vi "addDevices.vi"(0 "IDevice in":refnum<class "IDevice.lvclass">, 2 "Connection Arguments in":T1(c390), 3 "Error Codes in":map{string, refnum<class "IInteger.lvclass">}(c390), 4 "Error Infos in":map{string, refnum<class "IErrorInfo.lvclass">}(c390), 5 "error in (no error)":errorcluster) -> (14 "IDevice out":refnum<class "IDevice.lvclass">, 15 "Devices out":map{string, refnum<class "IDevice.lvclass">}(c390), 16 "Connection Arguments out":T1(c390), 17 "Error Codes out":map{string, refnum<class "IInteger.lvclass">}(c390), 18 "Error Infos out":map{string, refnum<class "IErrorInfo.lvclass">}(c390), 19 "error out":errorcluster)   [LabVIEW 2022 SP3, in "openDAQ.lvlib" / "IBaseObject.lvlib" / "IPropertyObject.lvlib" / "IComponent.lvlib" / "IFolder.lvlib" / "IDevice.lvlib" / "IDevice.lvclass"]
uses:
  <instrlib>/openDAQ/Public/Classes/IDevice/IDevice.lvclass
  <instrlib>/openDAQ/Public/Classes/IDevice/IDevice.lvclass/IDevice.ctl
  <instrlib>/openDAQ/Public/Classes/daqCoreTypes/IDict/IDict.lvclass
  <instrlib>/openDAQ/Binaries/Windows/x86/copendaq32.dll
  <instrlib>/openDAQ/Public/Classes/daqUtils/daqUtils.lvlib
  <instrlib>/openDAQ/Public/Classes/daqCoreTypes/IDict/Polymorphic/getValueList/getDeviceValueList.vi
  <instrlib>/openDAQ/Public/Classes/daqCoreTypes/IDict/Polymorphic/getKeyList/getStringKeyList.vi
  <instrlib>/openDAQ/Public/Classes/daqCoreTypes/IInteger/IInteger.lvclass
  <instrlib>/openDAQ/Public/Classes/IPropertyObject/IPropertyObject.lvclass
  <instrlib>/openDAQ/Public/Classes/IErrorInfo/IErrorInfo.lvclass
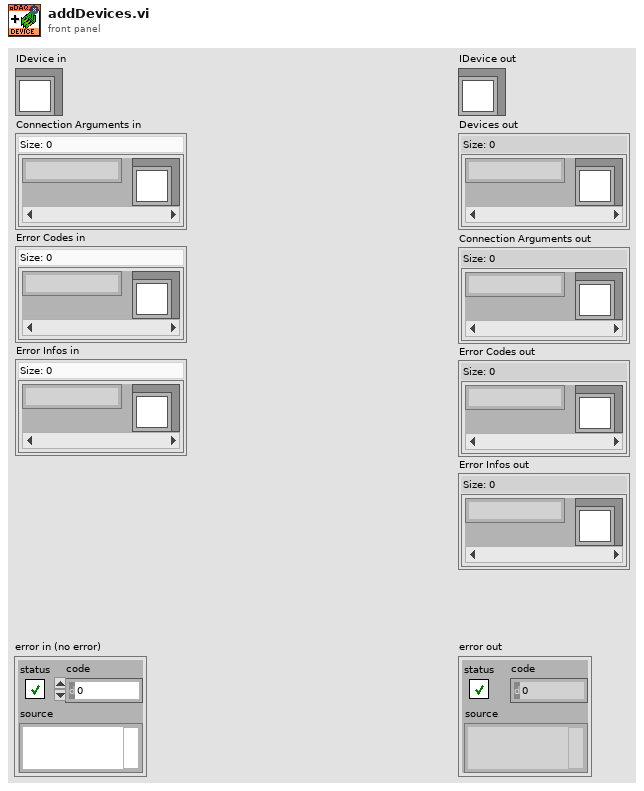
[diagram p1: front panel]
types:
  T1 = map{string, refnum<class "IPropertyObject.lvclass">}
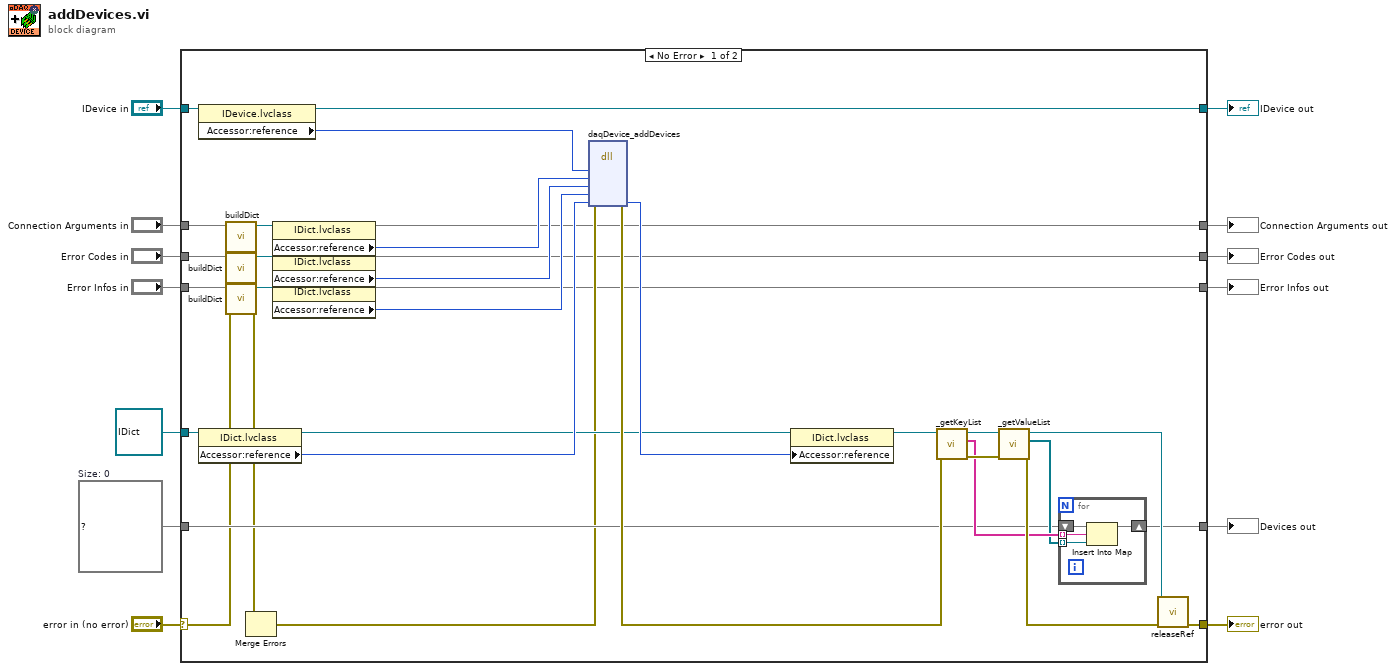
[diagram p0: block diagram]
diagram:
  w8 = map{string, refnum<class "IDevice.lvclass">} {}  # Size: 0
  n1 = case shown="No Error" "error in (no error)" {
    selector: "error in (no error)" -> [w27 w55]
    tunnel: [w34 w55] -> w12
    tunnel: [w41 w54] -> w10
    tunnel: "IDevice in" -> [w43 w54]
    tunnel: refnum<class "IDict.lvclass"> refnum ("openDAQ.lvlib:daqCoreTypes.lvlib:IDict.lvclass") -> [w40 _]
    tunnel: w8 -> [w30 w53]
    tunnel: [w29 w53] -> w7
    tunnel: "Error Codes in" -> [w15 w51]
    tunnel: "Connection Arguments in" -> [w16 w52]
    tunnel: "Error Infos in" -> [w14 w50]
    tunnel: [w16 w52] -> w3
    tunnel: [w15 w51] -> w2
    tunnel: [w14 w50] -> w1
    frame No Error {
      n2 = property class="IDevice.lvclass"(reference=w43) -> (reference out=w41:refnum<class "IDevice.lvclass">, "Accessor:reference"=w42:i64)  [unwired: 1 in, 1 out]
      n3 = property class="IDict.lvclass"(reference=w40) -> (reference out=w28:refnum<class "IDict.lvclass">, "Accessor:reference"=w39:i64)  [unwired: 1 in, 1 out]
      n4 = call <instrlib>:"buildDict.vi"("error in (no error)"=w27, "Map in"=w16) -> ("error out"=w24:errorcluster, "IDict out"=w22:refnum<class "IDict.lvclass">)  [unwired: 8 in]
      n5 = call <instrlib>:"buildDict.vi"("error in (no error)"=w27, "Map in"=w15) -> ("error out"=w25:errorcluster, "IDict out"=w21:refnum<class "IDict.lvclass">)  [unwired: 8 in]
      n6 = call <instrlib>:"buildDict.vi"("error in (no error)"=w27, "Map in"=w14) -> ("error out"=w26:errorcluster, "IDict out"=w20:refnum<class "IDict.lvclass">)  [unwired: 8 in]
      n7 = Merge Errors(w24, w25, w26) -> (w23:errorcluster)
      n8 = property class="IDict.lvclass"(reference=w22) -> ("Accessor:reference"=w19:i64)  [unwired: 1 in, 2 out]
      n9 = property class="IDict.lvclass"(reference=w21) -> ("Accessor:reference"=w18:i64)  [unwired: 1 in, 2 out]
      n10 = property class="IDict.lvclass"(reference=w20) -> ("Accessor:reference"=w17:i64)  [unwired: 1 in, 2 out]
      n11 = dll-call lib="C:/Program Files (x86)/National Instruments/LabVIEW 2022/instr.lib/openDAQ/Binaries/Windows/x86/copendaq*.*" fn="daqDevice_addDevices"(error in=w23, "device"=w42, "connectionArgs"=w19, "errcodes"=w18, "errorInfo"=w17, "devices"=w39) -> (error out=w45:errorcluster, "devices"=w44:i64)  [unwired: 7 in, 1 out]
      n12 = property class="IDict.lvclass"(reference=w28, "Accessor:reference"=w44) -> (reference out=w38:refnum<class "IDict.lvclass">)  [unwired: 1 in, 1 out]
      n13 = call-poly <instrlib>:"_getKeyList.vi"("error in (no error)"=w45, "IDict in"=w38) -> ("error out"=w36:errorcluster, "Key List out"=w32:string[], "IDict out"=w37:refnum<class "IDict.lvclass">)  [unwired: 7 in]
      n14 = call-poly <instrlib>:"_getValueList.vi"("error in (no error)"=w36, "IDict in"=w37) -> ("error out"=w35:errorcluster, "Devices out"=w31:refnum<class "IDevice.lvclass">[], "IDict out"=w33:refnum<class "IDict.lvclass">)  [unwired: 7 in]
      n15 = for {
        shift-right: [w46] -> w29
        shift-left: w30 -> [w49]
        tunnel: w32 -> [w48] mode=indexing
        tunnel: w31 -> [w47] mode=indexing
        n16 = Insert Into Map(map in=w49, key=w48, value=w47) -> (map out=w46:map{string, refnum<class "IDevice.lvclass">})  [unwired: 2 out]
      }
      n17 = call-dynamic "releaseRef.vi"("error in (no error)"=w35, "IBaseObject in"=w33) -> ("error out"=w34:errorcluster)  [unwired: 9 in]
    }
    frame Error {
    }
  }
  "error out" <- w12
  "IDevice out" <- w10
  "Devices out" <- w7
  "Connection Arguments out" <- w3
  "Error Codes out" <- w2
  "Error Infos out" <- w1
